vi "Zera_Motores-Set_Vel.vi"() -> ()   [LabVIEW 2014]
uses:
  <userlib>/Newport ESP301/Newport ESP301.lvlib
panel:
  out "Title":string="ALIGNMENT PROCEDURE"
  in  "Acceleration (0 units/s²)":dbl=1.0 min=0.0 format="%#.4g"
  in  "Velocity (units/s)":dbl=1.0 min=0.0 format="%#.4g"
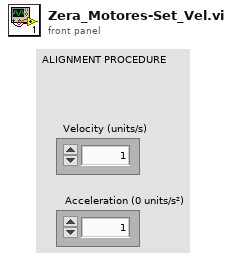
[diagram p1: front panel]
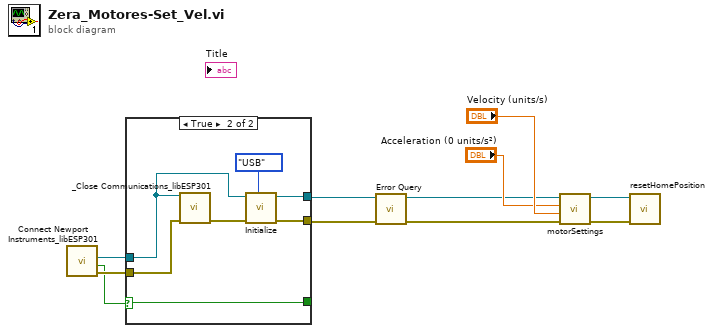
[diagram p0: block diagram]
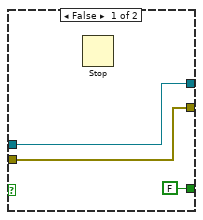
[diagram p2: hidden frame]
diagram:
  n1 = call <userlib>:"Connect Newport Instruments_libESP301.vi"() -> ("error (duplicate)"=w11:errorcluster, "Connected"=w7:bool, "VISA resource name (duplicate)"=w10:refnum<visa-resource-name>)  [unwired: 7 in, 2 out]
  n2 = case shown="True" w7 {
    selector: w7 -> [_ w15]
    tunnel: w11 -> [w12 w19]
    tunnel: w10 -> [w13 w18]
    tunnel: [w12 w17] -> w9
    tunnel: [w13 w16] -> w8
    tunnel: [FALSE w15] -> _
    frame False {
      n3 = Stop() -> ()  [unwired: 1 in]
    }
    frame True {
      n4 = call <userlib>:"_Close Communications_libESP301.vi"("Instrument Channel"=w18, "error in (no error)"=w19) -> ("error out"=w21:errorcluster)  [unwired: 13 in]
      n5 = call <userlib>:"Initialize.vi"("VISA resource name"=w18, "error in (no error)"=w21, "Serial Link (RS232)"=enum16{"RS232", "USB"}."USB") -> ("VISA resource name out"=w16:refnum<visa-resource-name>, "error out"=w17:errorcluster)  [unwired: 6 in]
    }
  }
  n6 = call <userlib>:"Error Query.vi"("error in (no error)"=w9, "VISA resource name"=w8) -> ("error out"=w1:errorcluster, "VISA resource name out"=w2:refnum<visa-resource-name>)  [unwired: 2 in, 2 out]
  n7 = call "motorSettings.vi"("error in (no error)"=w1, "Velocity (units/s)"="Velocity (units/s)", "Acceleration (0 units/s²)"="Acceleration (0 units/s²)", "VISA Refnum in"=w2) -> ("error out"=w3:errorcluster, "VISA Refnum out"=w4:refnum<visa-resource-name>)  [unwired: 6 in]
  n8 = call "resetHomePosition.vi"("error in (no error)"=w3, "VISA Refnum in"=w4) -> ()  [unwired: 8 in, 2 out]
